vi "XOR Encryption - (4) Key Rotation.vi"() -> ()   [LabVIEW 2016]
panel:
  out "Data Out":string[](array[string])
  in  "Data In":string[](array[string])
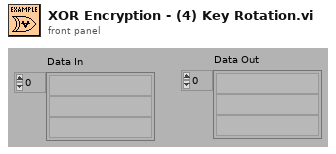
[diagram p1: front panel]
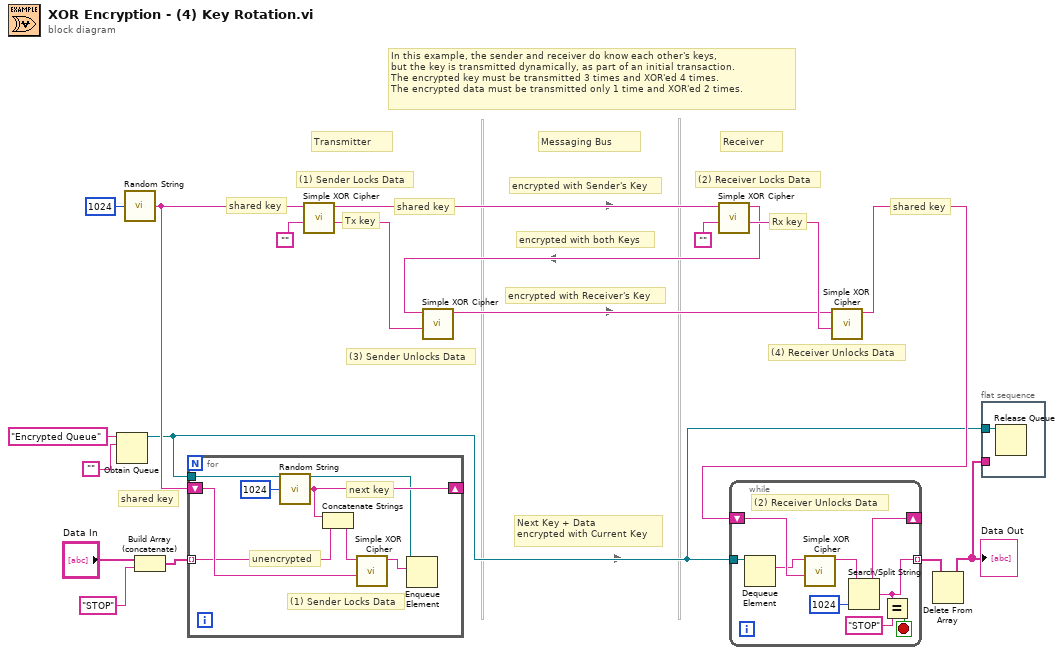
[diagram p0: block diagram]
diagram:
  # "shared key"
  # "shared key"
  # "shared key"
  # "Next Key + Data\nencrypted with Current Key"
  # "Messaging Bus"
  # "Receiver"
  # "Transmitter"
  # "shared key"
  # "Rx key"
  # "Tx key"
  # "In this example, the sender and receiver do know each other's keys,\nbut the key is transmitted dynamically, as part of an initial transaction.\nThe encrypted key must be transmitted 3 times and XOR'ed 4 times.\nThe encrypted data must be transmitted only 1 time and XOR'ed 2 times."
  # "encrypted with Receiver's Key"
  # "encrypted with Sender's Key"
  # "encrypted with both Keys"
  # "(4) Receiver Unlocks Data"
  # "(3) Sender Unlocks Data"
  # "(2) Receiver Locks Data"
  # "(1) Sender Locks Data"
  n1 = Obtain Queue(name (unnamed)="Encrypted Queue", element data type="") -> (queue out=w6:refnum<queue>)  [unwired: 3 in, 2 out]
  n2 = call "Random String.vi"("length"=1024) -> ("random data"=w10:string)  [unwired: 4 in]
  n3 = Build Array (concatenate)("Data In", "STOP" ("name (unnamed)")) -> (w4:string[])
  n4 = for {
    shift-right: [w22] -> _
    shift-left: w10 -> [w25]
    tunnel: w4 -> [w21] mode=indexing
    tunnel: w6 -> [w20]
    # "next key"
    # "unencrypted"
    # "(1) Sender Locks Data"
    n5 = call "Random String.vi"("length"=1024) -> ("random data"=w22:string)  [unwired: 4 in]
    n6 = Concatenate Strings(w22, w21) -> (w23:string)
    n7 = call "Simple XOR Cipher.vi"("key (\"\": random)"=w25, "data in"=w23) -> ("data out"=w19:string)  [unwired: 8 in, 1 out]
    n8 = Enqueue Element(queue=w20, element=w19) -> ()  [unwired: 2 in, 3 out]
  }
  n9 = call "Simple XOR Cipher.vi"("key (\"\": random)"="", "data in"=w10) -> ("key out"=w17:string, "data out"=w15:string)  [unwired: 8 in]
  n10 = call "Simple XOR Cipher.vi"("key (\"\": random)"="", "data in"=w15) -> ("key out"=w18:string, "data out"=w13:string)  [unwired: 8 in]
  n11 = call "Simple XOR Cipher.vi"("key (\"\": random)"=w17, "data in"=w13) -> ("data out"=w14:string)  [unwired: 8 in, 1 out]
  n12 = call "Simple XOR Cipher.vi"("key (\"\": random)"=w18, "data in"=w14) -> ("data out"=w9:string)  [unwired: 8 in, 1 out]
  n13 = while {
    tunnel: [w28] -> w2 mode=indexing
    tunnel: w6 -> [w33]
    shift-right: [w29] -> _
    shift-left: w9 -> [w34]
    stop <- w26 stop-if-true
    # "(2) Receiver Unlocks Data"
    n14 = Dequeue Element(queue=w33) -> (element=w32:string)  [unwired: 2 in, 3 out]
    n15 = call "Simple XOR Cipher.vi"("key (\"\": random)"=w34, "data in"=w32) -> ("data out"=w30:string)  [unwired: 8 in, 1 out]
    n16 = Search/Split String(string=w30, offset (0)=1024) -> (substring before match=w29:string, match + rest of string=w28:string)  [unwired: 1 in, 1 out]
    n17 = Equal?(x=w28, y="STOP") -> (x = y?=w26:bool)
  }
  n18 = Delete From Array(array=w2) -> (array with subset deleted=w1:string[])  [unwired: 2 in, 1 out]
  "Data Out" <- w1
  n19 = flat-sequence {
    tunnel: w6 -> [w35]
    tunnel: w1 -> [_]
    frame #0 {
      n20 = Release Queue(queue=w35) -> ()  [unwired: 2 in, 3 out]
    }
  }
